vi "CleanupStreamFolders.vi"(8 "error in (no error)":errorcluster) -> (0 "error out":errorcluster)   [LabVIEW 2017, in "FileManager.lvlib"]
uses:
  <vilib>/addons/InsightCM/Devices/Shared/Common/FileManager/FileManager.lvlib
  <vilib>/addons/InsightCM/Utilities/GlobalConfiguration/GlobalConfiguration.lvlib
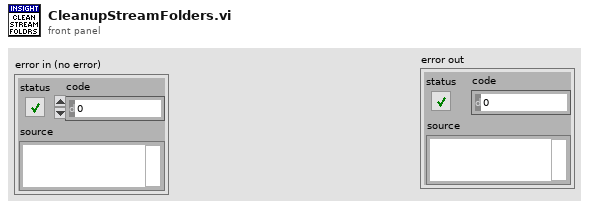
[diagram p1: front panel]
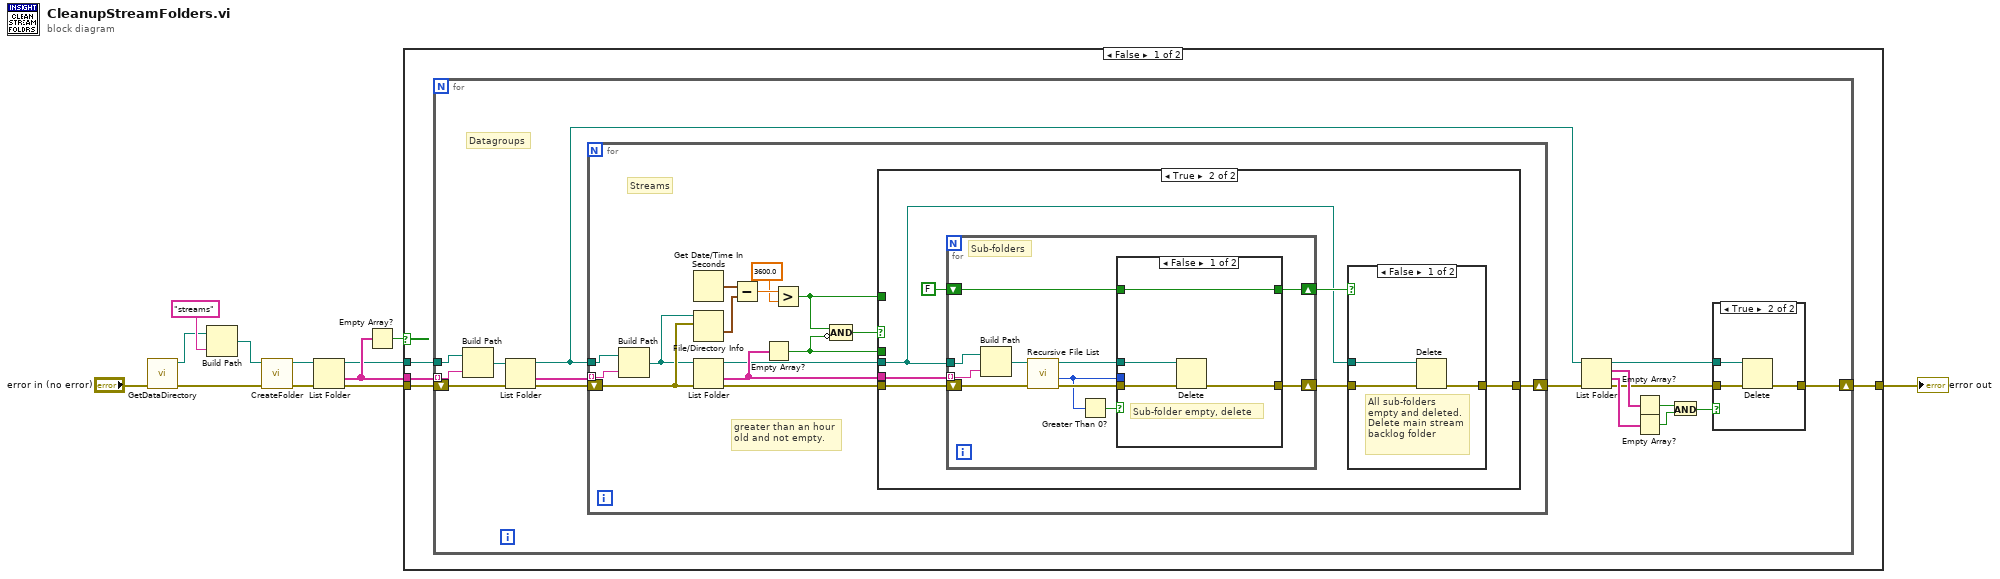
[diagram p0: block diagram]
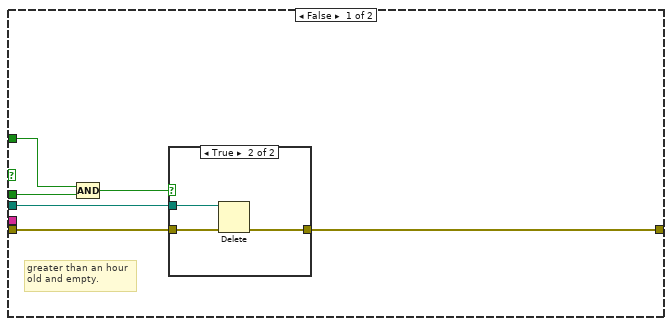
[diagram p3: hidden frame]
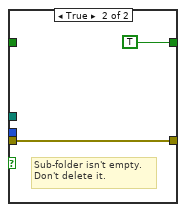
[diagram p5: hidden frame]
diagram:
  n1 = call <vilib>:"GetDataDirectory.vi"("error in (no error)"="error in (no error)") -> ("error out"=w8:errorcluster, "data directory"=w7:path)  [unwired: 9 in]
  n2 = Build Path(base path=w7, name or relative path="streams") -> (appended path=w10:path)
  n3 = call <vilib>:"CreateFolder.vi"("error in (no error)"=w8, "folder"=w10) -> ("error out"=w5:errorcluster, "folder out"=w6:path)  [unwired: 8 in]
  n4 = List Folder(path=w6, error in=w5) -> (path out=w1:path, folder names=w3:string[], error out=w4:errorcluster)  [unwired: 1 in, 2 out]
  n5 = Empty Array?(array=w3) -> (empty?=w2:bool)
  n6 = case shown="False" w2 {
    tunnel: [w16 w90] -> w12
    tunnel: w3 -> [w13 _]
    tunnel: w4 -> [w15 w90]
    tunnel: w1 -> [w14 _]
    frame False {
      n7 = for {
        shift-right: [w32] -> w16
        shift-left: w15 -> [w29]
        tunnel: w14 -> [w31]
        tunnel: w13 -> [w30] mode=indexing
        # "Datagroups"
        n8 = Build Path(base path=w31, name or relative path=w30) -> (appended path=w28:path)
        n9 = List Folder(path=w28, error in=w29) -> (path out=w26:path, folder names=w25:string[], error out=w27:errorcluster)  [unwired: 1 in, 2 out]
        n10 = for {
          tunnel: w25 -> [w49] mode=indexing
          tunnel: w26 -> [w50]
          shift-right: [w51] -> w24
          shift-left: w27 -> [w45]
          # "greater than an hour\nold and not empty."
          # "Streams"
          n11 = Build Path(base path=w50, name or relative path=w49) -> (appended path=w44:path)
          n12 = Get Date/Time In Seconds() -> (seconds since 1Jan1904=w43:timestamp)
          n13 = File/Directory Info(path=w44, error in=w45) -> (last mod=w42:timestamp)  [unwired: 6 out]
          n14 = List Folder(path=w44, error in=w45) -> (path out=w47:path, folder names=w48:string[], error out=w46:errorcluster)  [unwired: 1 in, 2 out]
          n15 = Subtract(x=w43, y=w42) -> (x-y=w41:dbl)
          n16 = Empty Array?(array=w48) -> (empty?=w38:bool)
          n17 = Greater?(x=w41, y=3600.0) -> (0:w37:bool)
          n18 = Compound Arithmetic op=AND(w37, invert w38) -> (w39:bool)
          n19 = case shown="True" w39 {
            tunnel: w46 -> [w53 w68]
            tunnel: [w52 w66] -> w51
            tunnel: w47 -> [w54 w62]
            tunnel: w48 -> [_ w63]
            tunnel: w38 -> [w57 _]
            tunnel: w37 -> [w56 _]
            frame False {
              # "greater than an hour\nold and empty."
              n20 = Compound Arithmetic op=AND(w56, w57) -> (w55:bool)
              n21 = case shown="True" w55 {
                tunnel: w54 -> [_ w61]
                tunnel: w53 -> [w58 w60]
                tunnel: [w58 w59] -> w52
                frame False {
                }
                frame True {
                  n22 = Delete(path (use dialog)=w61, error in=w60) -> (error out=w59:errorcluster)  [unwired: 3 in, 2 out]
                }
              }
            }
            frame True {
              n23 = for {
                shift-right: [w79] -> w67
                shift-left: w68 -> [w78]
                tunnel: w63 -> [w76] mode=indexing
                tunnel: w62 -> [w77]
                shift-right: [w69] -> w64
                shift-left: FALSE -> [w70]
                # "Sub-folders"
                n24 = Build Path(base path=w77, name or relative path=w76) -> (appended path=w75:path)
                n25 = call <vilib>:"Recursive File List.vi"("error in (no error)"=w78, "Folder Path"=w75) -> ("error out"=w74:errorcluster, "Number of Files"=w73:i32, "dup Folder Path"=w71:path)  [unwired: 5 in, 2 out]
                n26 = Greater Than 0?(x=w73) -> (x > 0?=w72:bool)
                n27 = case shown="False" w72 {
                  tunnel: [w82 w85] -> w79
                  tunnel: w74 -> [w83 w85]
                  tunnel: w73 -> [_ _]
                  tunnel: w71 -> [w81 _]
                  tunnel: w70 -> [w80 _]
                  tunnel: [w80 TRUE] -> w69
                  frame False {
                    # "Sub-folder empty, delete"
                    n28 = Delete(path (use dialog)=w81, error in=w83) -> (error out=w82:errorcluster)  [unwired: 3 in, 2 out]
                  }
                  frame True {
                    # "Sub-folder isn't empty.\nDon't delete it."
                  }
                }
              }
              n29 = case shown="False" w64 {
                tunnel: w67 -> [w88 w89]
                tunnel: [w87 w89] -> w66
                tunnel: w62 -> [w86 _]
                frame False {
                  # "All sub-folders\nempty and deleted.\nDelete main stream\nbacklog folder"
                  n30 = Delete(path (use dialog)=w86, error in=w88) -> (error out=w87:errorcluster)  [unwired: 3 in, 2 out]
                }
                frame True {
                }
              }
            }
          }
        }
        n31 = List Folder(path=w26, error in=w24) -> (path out=w17:path, filenames=w23:string[], folder names=w22:string[], error out=w21:errorcluster)  [unwired: 1 in, 1 out]
        n32 = Empty Array?(array=w23) -> (empty?=w19:bool)
        n33 = Empty Array?(array=w22) -> (empty?=w18:bool)
        n34 = And(x=w19, y=w18) -> (x .and. y?=w20:bool)
        n35 = case shown="True" w20 {
          tunnel: [w33 w36] -> w32
          tunnel: w21 -> [w33 w35]
          tunnel: w17 -> [_ w34]
          frame False {
          }
          frame True {
            n36 = Delete(path (use dialog)=w34, error in=w35) -> (error out=w36:errorcluster)  [unwired: 3 in, 2 out]
          }
        }
      }
    }
    frame True {
    }
  }
  "error out" <- w12
